vi "Oversample Input.vi"(9 "NSamples":u8, 11 "Channel":refnum<k21>) -> (3 "Output":fxp<+/-,36,9>)   [LabVIEW 2014]
uses:
  <vilib>/rvi/eio/common/nirviEmuTemplateMethod_errors.vi
  <vilib>/eio/EIONode/EIONode.xnode
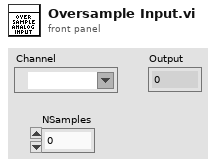
[diagram p1: front panel]
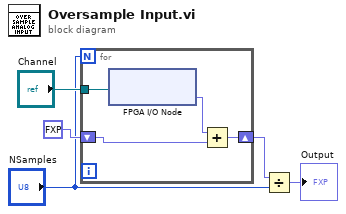
[diagram p0: block diagram]
diagram:
  n1 = for {
    N: "NSamples" -> [_]
    tunnel: "Channel" -> [w9]
    shift-right: [w8] -> w2
    shift-left: fxp<+/-,24,5> 0.0 ("I/O Item") -> [w6]
    n2 = xnode "FPGA I/O Node"("FPGA I/O In"=w9) -> ("I/O Item"=w7:fxp<+/-,24,5>)  [unwired: 1 out]
    n3 = Add(x=w7, y=w6) -> (x+y=w8:fxp<+/-,28,9>)
  }
  n4 = Divide(x=w2, y="NSamples") -> (x/y=→"Output":fxp<+/-,36,9>)
